vi "Get Gal Search Config.vi"(0 "Image":T1(plugin-control)) -> ()   [LabVIEW 2019]
uses:
  Framework/Robot Global Data.vi
  <vilib>/vision/NI_Vision_Development_Module.lvlib
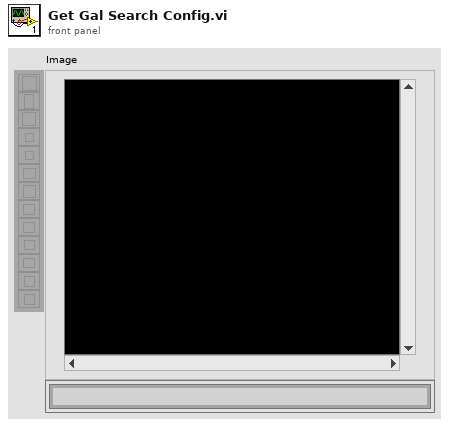
[diagram p1: front panel]
types:
  T1 = typedef "IMAQ Image.ctl" = refnum<image>
  T2 = typedef "Particle Parameters" = i32
  T3 = enum32{"AutoM", "Close", "Dilate", "Erode", "Gradient", "Gradient out", "Gradient in", "Hit miss", "Open", "PClose", "POpen", "Thick", "Thin"}
  T4 = typedef "Image Type" = u32
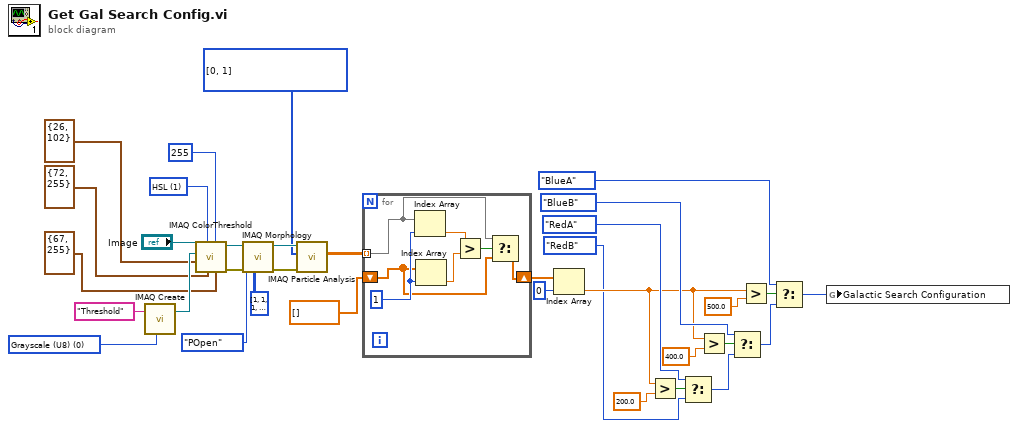
[diagram p0: block diagram]
diagram:
  w19 = T2[] [0, 1] items=["Center of Mass X", "Center of Mass Y", "First Pixel X", "First Pixel Y", "Bounding Rect Left", "Bounding Rect Top", "Bounding Rect Right", "Bounding Rect Bottom", "Max Feret Diameter Start X", "Max Feret Diameter Start Y", "Max Feret Diameter End X", "Max Feret Diameter End Y", "Max Horiz. Segment Length Left", "Max Horiz. Segment Length Right", "Max Horiz. Segment Length Row", "-", "Bounding Rect Width", "Bounding Rect Height", "Bounding Rect Diagonal", "Perimeter", "Convex Hull Perimeter", "Holes' Perimeter", "Max Feret Diameter", "Equivalent Ellipse Major Axis", "Equivalent Ellipse Minor Axis", "Equivalent Ellipse Minor Axis (Feret)", "Equivalent Rect Long Side", "Equivalent Rect Short Side", "Equivalent Rect Diagonal", "Equivalent Rect Short Side (Feret)", "Average Horiz. Segment Length", "Average Vert. Segment Length", "Hydraulic Radius", "Waddel Disk Diameter", "-", "Area", "Holes' Area", "Particle & Holes' Area", "Convex Hull Area", "Image Area", "-", "Number of Holes", "Number of Horiz. Segments", "Number of Vert. Segments", "-", "Orientation", "Max Feret Diameter Orientation", "-", "% Area/Image Area", "% Area/(Particle & Holes' Area)", "Ratio of Equivalent Ellipse Axes", "Ratio of Equivalent Rect Sides", "-", "Elongation Factor", "Compactness Factor", "Heywood Circularity Factor", "Type Factor", "-", "Sum X", "Sum Y", "Sum XX", "Sum XY", "Sum YY", "Sum XXX", "Sum XXY", "Sum XYY", "Sum YYY", "-", "Moment of Inertia XX", "Moment of Inertia XY", "Moment of Inertia YY", "Moment of Inertia XXX", "Moment of Inertia XXY", "Moment of Inertia XYY", "Moment of Inertia YYY", "Norm. Moment of Inertia XX", "Norm. Moment of Inertia XY", "Norm. Moment of Inertia YY", "Norm. Moment of Inertia XXX", "Norm. Moment of Inertia XXY", "Norm. Moment of Inertia XYY", "Norm. Moment of Inertia YYY", "Hu Moment 1", "Hu Moment 2", "Hu Moment 3", "Hu Moment 4", "Hu Moment 5", "Hu Moment 6", "Hu Moment 7"] ("Pixel Measurements")
  w31 = u16 1 items=["RGB", "HSL", "HSV", "HSI"] ("Color Mode")
  w27 = T4 0 items=["Grayscale (U8)", "Grayscale (I16)", "Grayscale (SGL)", "Complex (CSG)", "RGB (U32)", "HSL (U32)", "RGB (U64)", "Grayscale (U16)"] ("Image Type")
  n1 = call "IMAQ Create"("Image Name"="Threshold", "Image Type"=w27) -> ("New Image"=w32:T1)  [unwired: 3 in, 1 out]
  n2 = call "IMAQ ColorThreshold"("Blue or Luma or Val or Inten Range"=cluster{"Lower value":i32, "Upper value":i32} {"Lower value"=67, "Upper value"=255} ("Green or Sat Range"), "Replace Value"=255, "Green or Sat Range"=cluster{"Lower value":i32, "Upper value":i32} {"Lower value"=72, "Upper value"=255}, "Color Mode"=w31, "Red or Hue Range"=cluster{"Lower value":i32, "Upper value":i32} {"Lower value"=26, "Upper value"=102}, "Image Dst"=w32, "Image Src"="Image") -> ("error out"=w24:errorcluster, "Image Dst Out"=w25:T1)  [unwired: 3 in]
  n3 = call "IMAQ Morphology"("Structuring Element"=i32[][] [[1, 1, 1, 1, 1], [1, 1, 1, 1, 1], [1, 1, 1, 1, 1], [1, 1, 1, 1, 1], [1, 1, 1, 1, 1]], "error in (no error)"=w24, "Operation"=T3."POpen", "Image Src"=w25) -> ("error out"=w21:errorcluster, "Image Dst Out"=w20:T1)  [unwired: 6 in]
  n4 = call "IMAQ Particle Analysis"("error in (no error)"=w21, "Pixel Measurements"=w19, "Image"=w20) -> ("Particle Measurements (Pixels)"=w18:dbl[][])  [unwired: 3 in, 5 out]
  n5 = for {
    tunnel: w18 -> [w37] mode=indexing
    shift-right: [w35] -> w16
    shift-left: dbl[] [] ("Particle Measurements (Pixels)") -> [w36]
    w41 = 1 ("index")
    n6 = Index Array(array=w37, index=w41) -> (element=w39:dbl)
    n7 = Index Array(array=w36, index=w41) -> (element=w40:dbl)
    n8 = Greater?(x=w39, y=w40) -> (0:w38:bool)
    n9 = Select(t=w37, s=w38, f=w36) -> (s? t:f=w35:dbl[])
  }
  n10 = Index Array(array=w16, index=0) -> (element=w3:dbl)
  n11 = Greater?(x=w3, y=200.0) -> (0:w6:bool)
  n12 = Select(t=enum16{"RedA", "BlueA", "RedB", "BlueB"}."RedA" ("Galactic Search Configuration"), s=w6, f=enum16{"RedA", "BlueA", "RedB", "BlueB"}."RedB" ("Galactic Search Configuration")) -> (s? t:f=w7:enum16{"RedA", "BlueA", "RedB", "BlueB"})
  n13 = Greater?(x=w3, y=400.0) -> (0:w10:bool)
  n14 = Select(t=enum16{"RedA", "BlueA", "RedB", "BlueB"}."BlueB" ("Galactic Search Configuration"), s=w10, f=w7) -> (s? t:f=w9:enum16{"RedA", "BlueA", "RedB", "BlueB"})
  n15 = Greater?(x=w3, y=500.0) -> (0:w13:bool)
  n16 = Select(t=enum16{"RedA", "BlueA", "RedB", "BlueB"}."BlueA" ("Galactic Search Configuration"), s=w13, f=w9) -> (s? t:f=w1:enum16{"RedA", "BlueA", "RedB", "BlueB"})
  n17 = global write "Robot Global Data.vi" "Galactic Search Configuration"(w1) -> ()
